vi "NEW Set Drive Motors.vi"(5 "Disable":bool, 7 "Max Velocity(RPM)":dbl=200.0, 8 "Control Mode":T3 items=["PercentOutput"=0, "Position"=1, "Velocity"=2, "Current"=3, "Follower"=5, "MotionProfile"=6, "MotionMagic"=7, "MotionProfileArc"=10, "Disabled"=15], 9 "Specific Module Data":T1[](array[typedef])=[{"Motor Pos"=enum."Left-Front", "CAN Bus"="", "Drive ID"=5, "Azimuth ID"=1, "CanCoder ID"=1, "CanCoder Offset"=283.711}, {"Motor Pos"=enum."Right-Front", "CAN Bus"="", "Drive ID"=6, "Azimuth ID"=2, "CanCoder ID"=2, "CanCoder Offset"=79.695}, {"Motor Pos"=enum."Right-Back", "CAN Bus"="", "Drive ID"=7, "Azimuth ID"=3, "CanCoder ID"=3, "CanCoder Offset"=319.746}, {"Motor Pos"=enum."Left-Back", "CAN Bus"="", "Drive ID"=7, "Azimuth ID"=3, "CanCoder ID"=3, "CanCoder Offset"=319.746}], 10 "Swerve Data":T4 {"Back Right"."Angle" scale format="%.3f"; "Back Right"."Velocity" scale=-1.0..1.0 scale format="%.1f"; "Back Left"."Angle" scale format="%.3f"; "Back Left"."Velocity" scale=-1.0..1.0 scale format="%.1f"; "Front Left"."Angle" scale format="%.3f"; "Front Left"."Velocity" scale=-1.0..1.0 scale format="%.1f"; "Front Right"."Angle" scale format="%.3f"; "Front Right"."Velocity" scale=-1.0..1.0 scale format="%.1f"}, 11 "Drive Refs":T8[](array[typedef])) -> (1 "Speeds":dbl[](array[numeric]), 3 "Array Out":T8[](array[typedef]))   [LabVIEW 2020, in "SwerveDrive_ACT.lvlib"]
uses:
  SwerveDrive_ACT.lvlib
  <vilib>/Rock Robotics/WPI/MotorControl/WPI_MotorControlDeviceRef.ctl
  <vilib>/Rock Robotics/WPI/MotorControl/WPI_MotorControlType.ctl
  <vilib>/Rock Robotics/SystemInterfaces/DIO/FPGA_DIOPWMChannel.ctl
  <vilib>/Rock Robotics/WPI/PWM/WPI_PWMDeadband.ctl
  <vilib>/Rock Robotics/SystemInterfaces/DIO/FPGA_DIOChannel.ctl
  Shared Code/TypeDefs/Cluster_Swerve 4 Steer and Velocity.ctl
  Shared Code/TypeDefs/Cluster_Module Velocity-Direction-Rotations.ctl
  Shared Code/TypeDefs/Level_Velocity plus-minus 1.ctl
  Shared Code/TypeDefs/Dial_Compase heading unit circle CCW positive.ctl
  <vilib>/Rock Robotics/WPI/ThirdParty/Phoenix-LabVIEW/Motor Controller/Controls/CTRE_Phoenix_MotorControl_ControlMode.ctl
  Shared Code/TypeDefs/Cluster_Module Specific Config Data.ctl
  Shared Code/TypeDefs/ENUM_Motor Index.ctl
panel:
  # "\"Front\" of Robot"
  # "Right Hand Rule"
  # "X"
  # "+CCW"
  # "Y"
  # "(0,0)"
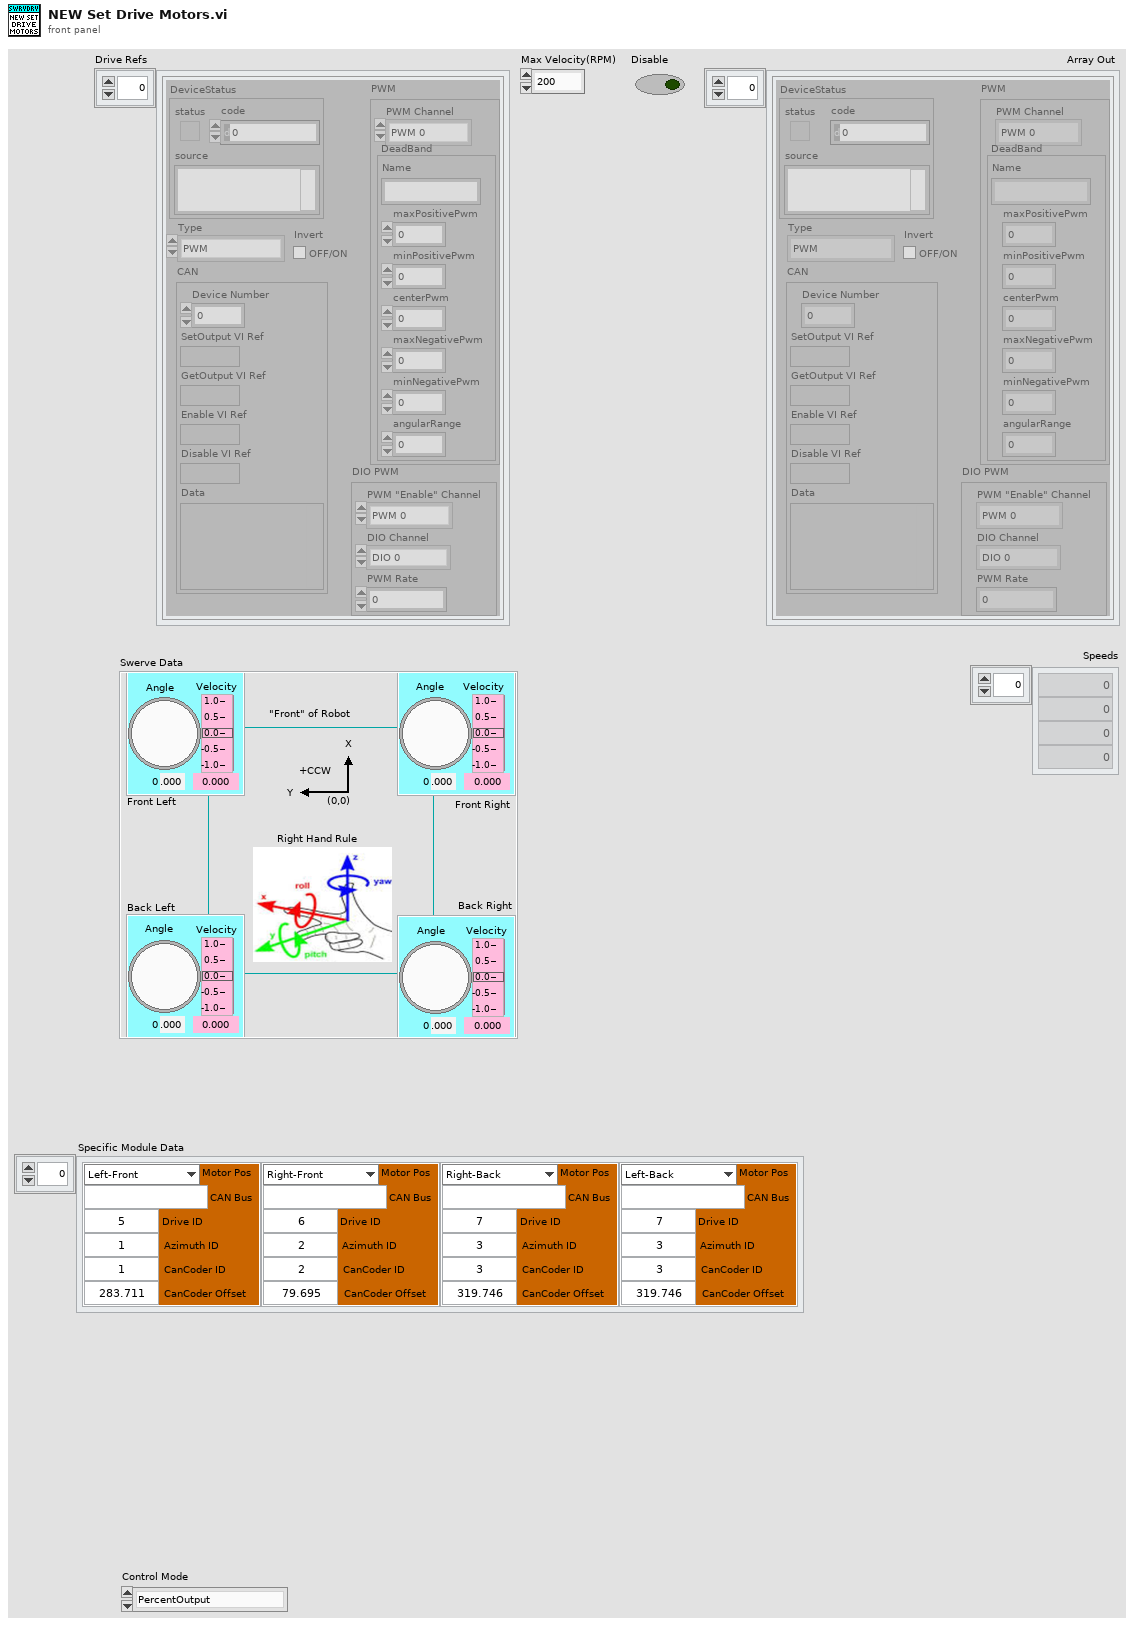
[diagram p1: front panel]
types:
  T1 = typedef "Cluster_Module Specific Config Data.ctl" = cluster{"Motor Pos":T2, "CAN Bus":string, "Drive ID":u8, "Azimuth ID":u8, "CanCoder ID":u8, "CanCoder Offset":dbl}
  T2 = typedef "ENUM_Motor Index.ctl" = enum16{"Left-Front", "Right-Front", "Left-Back", "Right-Back"}
  T3 = typedef "CTRE_Phoenix_MotorControl_ControlMode.ctl" = u16
  T4 = typedef "Cluster_Swerve 4 Steer and Velocity.ctl" = cluster{"Front Right":T5, "Front Left":T5, "Back Left":T5, "Back Right":T5}
  T5 = typedef "Cluster_Module Velocity-Direction-Rotations.ctl" = cluster{"Velocity":T6, "Angle":T7, "Rotations Count":dbl}
  T6 = typedef "Level_Velocity plus-minus 1.ctl" = dbl
  T7 = typedef "Dial_Compase heading unit circle CCW positive.ctl" = dbl
  T8 = typedef "WPI_MotorControlDeviceRef.ctl" = cluster{"DeviceStatus":errorcluster, "Type":T9, "PWM":cluster{"PWM Channel":T10, "DeadBand":T11}, "CAN":cluster{"Device Number":u8, "SetOutput VI Ref":variant, "GetOutput VI Ref":variant, "Enable VI Ref":variant, "Disable VI Ref":variant, "Data":variant}, "Invert":bool, "DIO PWM":cluster{"PWM \"Enable\" Channel":T10, "DIOChannel":T12, "PWM Rate":dbl}}
  T9 = typedef "WPI_MotorControlType.ctl" = enum16{"PWM", "CAN", "DIO PWM"}
  T10 = typedef "FPGA_DIOPWMChannel.ctl" = enum8{"PWM 0", "PWM 1", "PWM 2", "PWM 3", "PWM 4", "PWM 5", "PWM 6", "PWM 7", "PWM 8", "PWM 9", "PWM MXP 0", "PWM MXP 1", "PWM MXP 2", "PWM MXP 3", "PWM MXP 4", "PWM MXP 5", "PWM MXP 6", "PWM MXP 7", "PWM MXP 8", "PWM MXP 9", "Invalid"}
  T11 = typedef "WPI_PWMDeadband.ctl" = cluster{"Name":string, "maxPositivePwm":i32, "minPositivePwm":i32, "centerPwm":i32, "maxNegativePwm":i32, "minNegativePwm":i32, "angularRange":u16}
  T12 = typedef "FPGA_DIOChannel.ctl" = enum8{"DIO 0", "DIO 1", "DIO 2", "DIO 3", "DIO 4", "DIO 5", "DIO 6", "DIO 7", "DIO 8", "DIO 9", "DIO MXP 0", "DIO MXP 1", "DIO MXP 2", "DIO MXP 3", "DIO MXP 4", "DIO MXP 5", "DIO MXP 6", "DIO MXP 7", "DIO MXP 8", "DIO MXP 9", "DIO MXP 10", "DIO MXP 11", "DIO MXP 12", "DIO MXP 13", "DIO MXP 14", "DIO MXP 15", "SPI Port CS1", "SPI Port CS2", "SPI Port CS3", "SPI Port MISO", "SPI Port MOSI", "Invalid"}
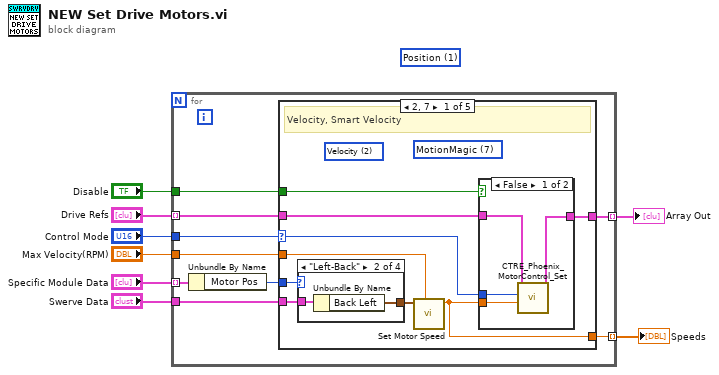
[diagram p0: block diagram]
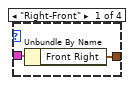
[diagram p3: hidden frame]
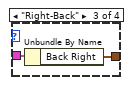
[diagram p4: hidden frame]
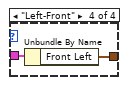
[diagram p5: hidden frame]
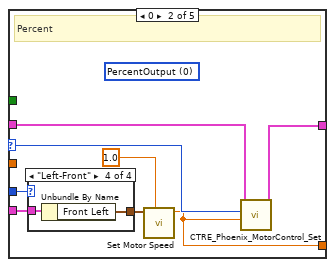
[diagram p6: hidden frame]
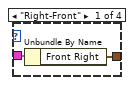
[diagram p7: hidden frame]
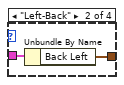
[diagram p8: hidden frame]
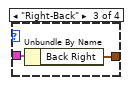
[diagram p9: hidden frame]
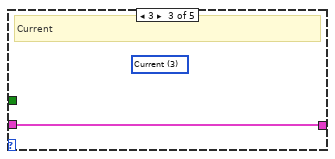
[diagram p10: hidden frame]
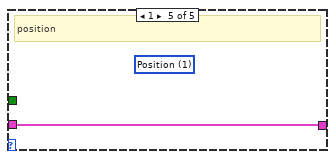
[diagram p12: hidden frame]
diagram:
  (unwired) T3 1 items=["PercentOutput"=0, "Position"=1, "Velocity"=2, "Current"=3, "Follower"=5, "MotionProfile"=6, "MotionMagic"=7, "MotionProfileArc"=10, "Disabled"=15] ("Control Mode")
  n1 = for {
    tunnel: "Drive Refs" -> [w17] mode=indexing
    tunnel: "Control Mode" -> [w16]
    tunnel: [w15] -> w8 mode=indexing
    tunnel: "Max Velocity(RPM)" -> [w12]
    tunnel: "Specific Module Data" -> [w14] mode=indexing
    tunnel: "Swerve Data" -> [w13]
    tunnel: [w11] -> w4 mode=indexing
    tunnel: "Disable" -> [w10]
    n2 = Unbundle By Name(w14) -> ("Motor Pos"=w9:T2)
    n3 = case shown="2, 7" w16 {
      selector: w16 -> [w25 w46 _ _ _]
      tunnel: w17 -> [w26 w47 w56 w57 w58]
      tunnel: [w24 w45 w56 w57 w58] -> w15
      tunnel: w9 -> [w22 w43 _ _ _]
      tunnel: w13 -> [w23 w44 _ _ _]
      tunnel: w12 -> [w20 _ _ _ _]
      tunnel: [w19 w40 _ _ _] -> w11
      tunnel: w10 -> [w18 _ _ _ _]
      frame 2, 7 {
        (unwired) T3 7 items=["PercentOutput"=0, "Position"=1, "Velocity"=2, "Current"=3, "Follower"=5, "MotionProfile"=6, "MotionMagic"=7, "MotionProfileArc"=10, "Disabled"=15] ("Control Mode")
        (unwired) T3 2 items=["PercentOutput"=0, "Position"=1, "Velocity"=2, "Current"=3, "Follower"=5, "MotionProfile"=6, "MotionMagic"=7, "MotionProfileArc"=10, "Disabled"=15] ("Control Mode")
        # "Velocity, Smart Velocity"
        n4 = case shown="\"Left-Back\"" w22 {
          tunnel: w23 -> [w33 w35 w37 w39]
          tunnel: [w32 w34 w36 w38] -> w21
          frame "Right-Front" {
            n5 = Unbundle By Name(w33) -> ("Front Right"=w32:T5)
          }
          frame "Left-Back" {
            n6 = Unbundle By Name(w35) -> ("Back Left"=w34:T5)
          }
          frame "Right-Back" {
            n7 = Unbundle By Name(w37) -> ("Back Right"=w36:T5)
          }
          frame "Left-Front" {
            n8 = Unbundle By Name(w39) -> ("Front Left"=w38:T5)
          }
        }
        n9 = call "Set Motor Speed.vi"("Max Velocity"=w20, "Front Left"=w21) -> ("Velocity Value Set Out"=w19:dbl)  [unwired: 9 in]
        n10 = case shown="False" w18 {
          tunnel: w26 -> [w30 w31]
          tunnel: w25 -> [w27 _]
          tunnel: [w29 w31] -> w24
          tunnel: w19 -> [w28 _]
          frame False {
            n11 = call <vilib>:"CTRE_Phoenix_MotorControl_Set.vi"("Output"=w28, "Control Mode"=w27, "PhoenixMotorControlDevRef"=w30) -> ("PhoenixMotorControlDevRef"=w29:T8)  [unwired: 7 in, 1 out]
          }
          frame True {
          }
        }
      }
      frame 0 {
        (unwired) T3 0 items=["PercentOutput"=0, "Position"=1, "Velocity"=2, "Current"=3, "Follower"=5, "MotionProfile"=6, "MotionMagic"=7, "MotionProfileArc"=10, "Disabled"=15] ("Control Mode")
        # "Percent"
        n12 = case shown="\"Left-Front\"" w43 {
          tunnel: w44 -> [w49 w51 w53 w55]
          tunnel: [w48 w50 w52 w54] -> w42
          frame "Right-Front" {
            n13 = Unbundle By Name(w49) -> ("Front Right"=w48:T5)
          }
          frame "Left-Back" {
            n14 = Unbundle By Name(w51) -> ("Back Left"=w50:T5)
          }
          frame "Right-Back" {
            n15 = Unbundle By Name(w53) -> ("Back Right"=w52:T5)
          }
          frame "Left-Front" {
            n16 = Unbundle By Name(w55) -> ("Front Left"=w54:T5)
          }
        }
        n17 = call "Set Motor Speed.vi"("Max Velocity"=1.0, "Front Left"=w42) -> ("Velocity Value Set Out"=w40:dbl)  [unwired: 9 in]
        n18 = call <vilib>:"CTRE_Phoenix_MotorControl_Set.vi"("Output"=w40, "Control Mode"=w46, "PhoenixMotorControlDevRef"=w47) -> ("PhoenixMotorControlDevRef"=w45:T8)  [unwired: 7 in, 1 out]
      }
      frame 3 {
        (unwired) T3 3 items=["PercentOutput"=0, "Position"=1, "Velocity"=2, "Current"=3, "Follower"=5, "MotionProfile"=6, "MotionMagic"=7, "MotionProfileArc"=10, "Disabled"=15] ("Control Mode")
        # "Current"
      }
      frame Default {
      }
      frame 1 {
        (unwired) T3 1 items=["PercentOutput"=0, "Position"=1, "Velocity"=2, "Current"=3, "Follower"=5, "MotionProfile"=6, "MotionMagic"=7, "MotionProfileArc"=10, "Disabled"=15] ("Control Mode")
        # "position"
      }
    }
  }
  "Array Out" <- w8
  "Speeds" <- w4
